vi "test-PID-generateData.vi"(8 "error in (no error)":errorcluster) -> (0 "error out":errorcluster)   [LabVIEW 2019]
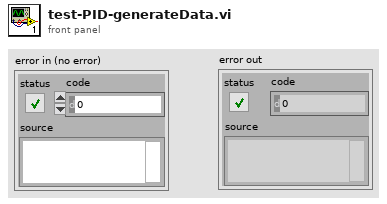
[diagram p1: front panel]
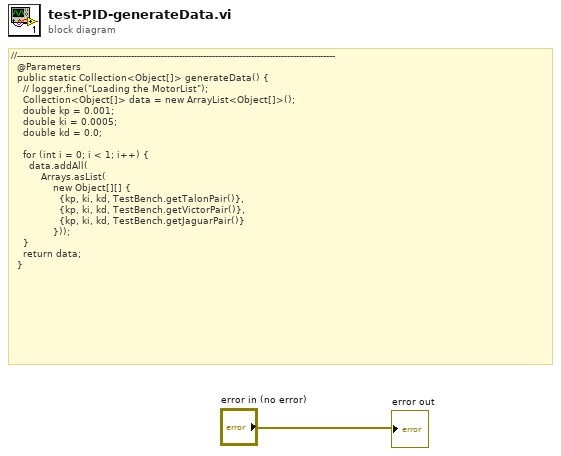
[diagram p0: block diagram]
diagram:
  # "//----------------------------------------------------------------------------------------------------------\n  @Parameters\n  public static Collection<Object[]> generateData() {\n    // logger.fine(\"Loading the MotorList\");\n    Collection<Object[]> data = new ArrayList<Object[]>();\n    double kp = 0.001;\n    double ki = 0.0005;\n    double kd = 0.0;\n\n    for (int i = 0; i < 1; i++) {\n      data.addAll(\n          Arrays.asList(\n              new Object[][] {\n                {kp, ki, kd, TestBench.getTalonPair()},\n                {kp, ki, kd, TestBench.getVictorPair()},\n                {kp, ki, kd, TestBench.getJaguarPair()}\n              }));\n    }\n    return data;\n  }"
  "error out" <- "error in (no error)"
